vi "FTW-JSON-Object-GetElement-String.vi"(0 "JSON Object":refnum<data-value>, 5 "Key":string, 7 "Default Value":string, 11 "error in":errorcluster) -> (4 "JSON Object out":refnum<data-value>, 8 "Value":string, 10 "Found?":bool, 15 "error out":errorcluster)   [LabVIEW 2014]
uses:
  core/FTW-JSON-Core-Structure.ctl
  error/FTW-ERR-ThrowGenericError.vi
  error/FTW-ERR-ThrowError.vi
  error/FTW-ERR-NoErrorConstant.vi
  error/FTW-ERR-CallChain.vi
  string/FTW-STR-ReplaceWhitespace.vi
panel:
  # "Inputs"
  # "Outputs"
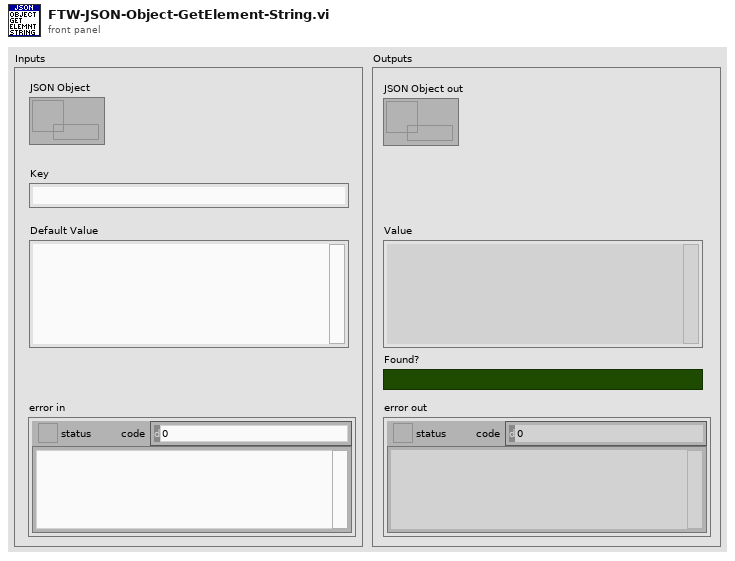
[diagram p1: front panel]
types:
  T1 = typedef "FTW-JSON-Core-Structure.ctl" = cluster{"JSON Object":i64, "Encoding Flags":i64, "Decoding Flags":i64}
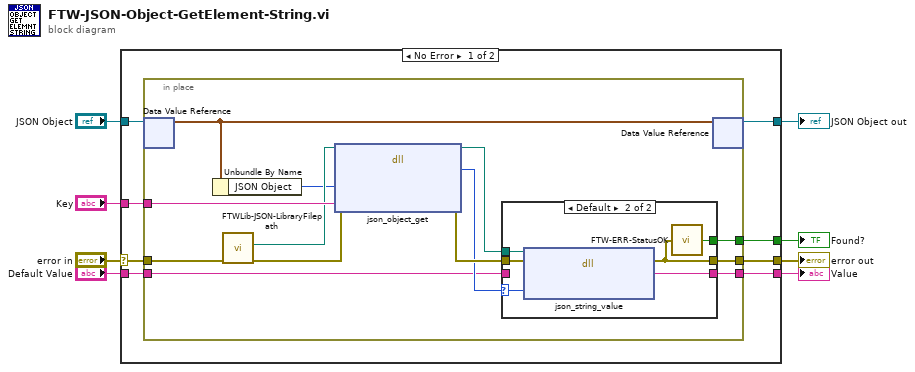
[diagram p0: block diagram]
diagram:
  n1 = case shown="No Error" "error in" {
    selector: "error in" -> [w16 w40]
    tunnel: [w14 w40] -> w8
    tunnel: [w9 w39] -> w6
    tunnel: "JSON Object" -> [w10 w39]
    tunnel: "Key" -> [w15 _]
    tunnel: [w13 w38] -> w2
    tunnel: [w12 _] -> w4
    tunnel: "Default Value" -> [w11 w38]
    frame No Error {
      n2 = in-place {
        in-place-border: w16 -> [w29]
        in-place-border: w15 -> [w28]
        in-place-border: [w25] -> w14
        in-place-border: [w24] -> w13
        in-place-border: [w23] -> w12
        in-place-border: w11 -> [w19]
        n3 = in-place-dvr #1(w10) -> (w18:T1)  [unwired: 1 out]
        n4 = Unbundle By Name(w18) -> ("JSON Object"=w17:i64)
        n5 = call "FTWLib-JSON-LibraryFilepath.vi"("error in"=w29) -> ("error out"=w27:errorcluster, "JSON Library Filepath"=w26:path)  [unwired: 9 in]
        n6 = dll-call lib="?" fn="json_object_get"(path in=w26, error in=w27, "JSON Object Pointer"=w17, "Element Key"=w28) -> (path out=w21:path, error out=w22:errorcluster, "JSON Element Pointer"=w20:i64)  [unwired: 3 in]
        n7 = case shown="Default" w20 {
          selector: w20 -> [_ w34]
          tunnel: w22 -> [w31 w37]
          tunnel: [w31 w33] -> w25
          tunnel: [w30 w36] -> w24
          tunnel: w21 -> [_ w35]
          tunnel: [_ w32] -> w23
          tunnel: w19 -> [w30 _]
          frame 0 {
          }
          frame Default {
            n8 = dll-call lib="?" fn="json_string_value"(path in=w35, error in=w37, "JSON Element Pointer"=w34) -> (error out=w33:errorcluster, "String Value"=w36:string)  [unwired: 2 in, 1 out]
            n9 = call "FTW-ERR-StatusOK.vi"("error to check"=w33) -> ("Status OK?"=w32:bool)
          }
        }
        n10 = in-place-dvr #1(w18) -> (w9:refnum<data-value>)  [unwired: 1 out]
      }
    }
    frame Error {
    }
  }
  "error out" <- w8
  "JSON Object out" <- w6
  "Found?" <- w4
  "Value" <- w2
